vi "Msg.vi"(7 "LVCAM in":refnum<class "LVCAM.lvclass">, 11 "LVCAM Create Nest Msg in":refnum<class "LVCAM Create Nest Msg.lvclass">) -> (0 "error out":errorcluster, 2 "Destroyed Self?":bool, 5 "LVCAM out":refnum<class "LVCAM.lvclass">)   [LabVIEW 2021, in "LVCAM Create Nest.lvlib" / "LVCAM Create Nest Msg.lvclass"]
uses:
  LVCAM Create Nest Msg.lvclass
  LVCAM/LVCAM/LVCAM.lvclass
  LVCAM Create Nest/LVCAM Create Nest.lvclass
  LVCAM Create Nest Msg.lvclass/LVCAM Create Nest Msg.ctl
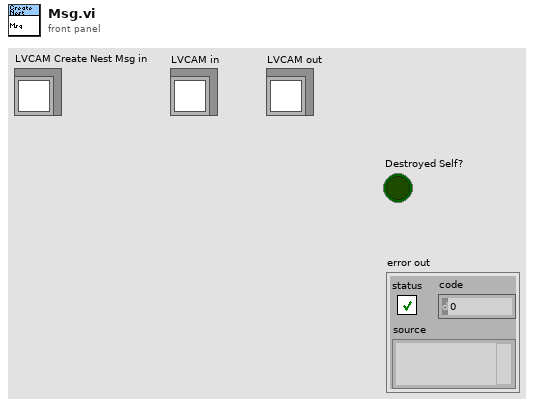
[diagram p1: front panel]
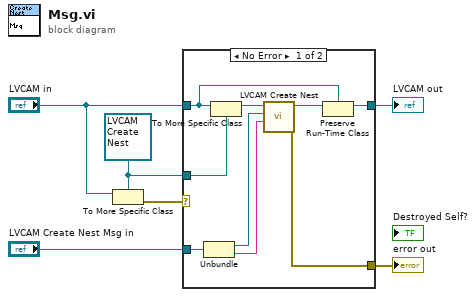
[diagram p0: block diagram]
diagram:
  w3 = refnum<class "LVCAM Create Nest.lvclass"> refnum ("Create.lvlib:Create.lvclass")
  n1 = To More Specific Class(target class=w3, reference="LVCAM in") -> (error out=w6:errorcluster)  [unwired: 1 in, 1 out]
  n2 = case shown="No Error" w6 {
    selector: w6 -> [_ w17]
    tunnel: [w13 w17] -> w4
    tunnel: [w8 w16] -> w2
    tunnel: "LVCAM in" -> [w7 w16]
    tunnel: "LVCAM Create Nest Msg in" -> [w12 _]
    tunnel: w3 -> [w10 _]
    frame No Error {
      n3 = Unbundle(w12) -> (w14:refnum<class "LVCAM.lvclass">, w15:string)
      n4 = To More Specific Class(target class=w10, reference=w7) -> (specific class reference=w11:refnum<class "LVCAM Create Nest.lvclass">)  [unwired: 1 in, 1 out]
      n5 = call-dynamic "LVCAM Create Nest.vi"("Alias"=w15, "Nest Actor"=w14, "LVCAM Create Nest in"=w11) -> ("error out"=w13:errorcluster, "LVCAM Create Nest out"=w9:refnum<class "LVCAM Create Nest.lvclass">)  [unwired: 7 in]
      n6 = Preserve Run-Time Class(object in=w9, 2:w7) -> (object out=w8:refnum<class "LVCAM.lvclass">)  [unwired: 1 in, 1 out]
    }
    frame Error {
    }
  }
  "error out" <- w4
  "LVCAM out" <- w2
